vi "Controller Write PS Setpoints.vi"(0 "PS Setpoint Variables":refnum<k21>[](array[refnum]), 1 "PS Enable Variables":refnum<k21>[](array[refnum]), 2 "PS Setpoints":dbl[](array[numeric]), 3 "error in (no error)":errorcluster) -> (10 "error out":errorcluster)   [LabVIEW 2011, in "Controller VIs.lvlib"]
doc: "Writes PS Setpoints variables to the Actuation chassis."
uses:
  Controller VIs.lvlib
  Simulated Beam VIs/Simulated PS Current.vi
  Simulated Beam VIs.lvlib
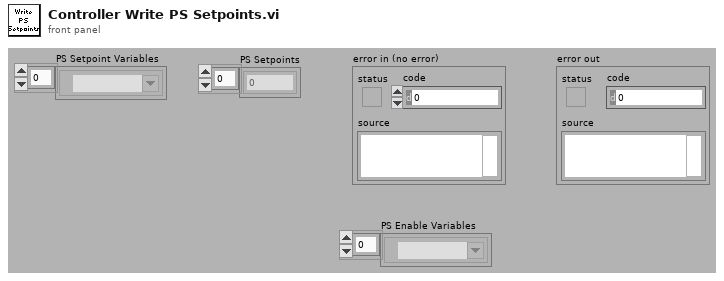
[diagram p1: front panel]
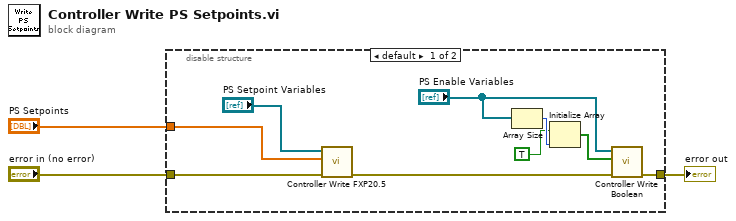
[diagram p0: block diagram]
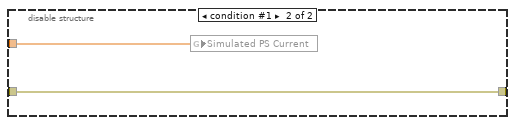
[diagram p2: hidden frame]
diagram:
  n1 = disable-structure shown="default" {
    disable-tunnel: "error in (no error)" -> [w12 w13]
    disable-tunnel: "PS Setpoints" -> [w10 w14]
    disable-tunnel: [w5 w13] -> w1
    frame condition #0 (active) {
      n2 = call "Controller Write FXP20.5.vi"("Error In"=w12, "Values"=w10, "Variables"="PS Setpoint Variables") -> ("Error Out"=w6:errorcluster)  [unwired: 8 in]
      n3 = Array Size(array="PS Enable Variables") -> (size(s)=w9:i32)
      n4 = Initialize Array(TRUE, w9) -> (w8:bool[])
      n5 = call "Controller Write Boolean.vi"("Error In"=w6, "Values"=w8, "Variables"="PS Enable Variables") -> ("Error Out"=w5:errorcluster)  [unwired: 8 in]
    }
    frame condition #1 {
      n6 = global write "Simulated PS Current.vi" "Simulated PS Current"(w14) -> ()
    }
  }
  "error out" <- w1
